vi "FestoCPX.Valve(2out2in).vi"(4 "Delay [ms] (0)":u32, 6 "Timeout [ms] (5000)":u32=5000, 8 "error in (no error)":errorcluster, 9 "Position":T3, 10 "Valve outputs":T1[](array[typedef]), 11 "Inputs":T2[](array[typedef])) -> (0 "error out":errorcluster, 2 "Aborted?":bool, 3 "Timeout?":bool)   [LabVIEW 2016]
uses:
  Station/Station.ValvePosition.ctl
  FestoCPX.DI.Signal.ctl
  FestoCPX.DO.Signal.ctl
  FestoCPX.DI.Data.State.Get.vi
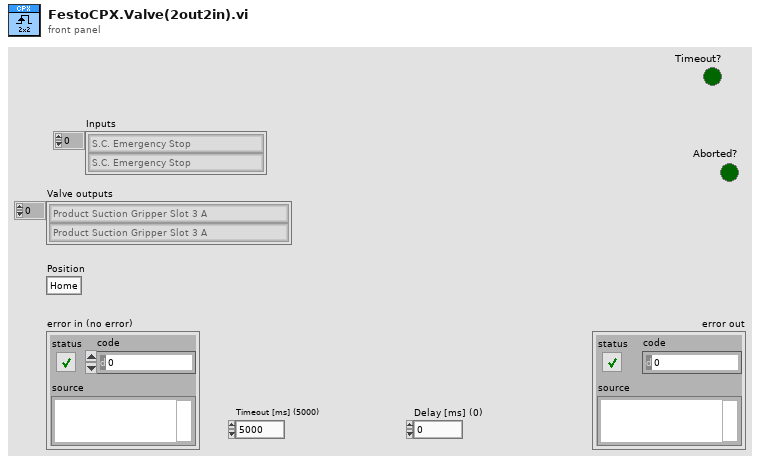
[diagram p1: front panel]
types:
  T1 = typedef "FestoCPX.DO.Signal.ctl" = enum16{"Safety Reset", "Air Main Valve", "Door Lock", "Button LED Start", "Button LED Stop", "Button LED Control", "Traffic LED Red", "Traffic LED Orange", "Traffic LED Green", "Horn", "Laser Interlock", "Laser Trigger", "Laser Fume Extractor", "Product Suction Gripper Slot 1 A", "Product Suction Gripper Slot 1 B", "Product Suction Gripper Slot 2 A", "Product Suction Gripper Slot 2 B", "Product Suction Gripper Slot 3 A", "Product Suction Gripper Slot 3 B", "Product Suction Gripper Slot 4 A", "Product Suction Gripper Slot 4 B", "Product Suction Gripper Final A", "Product Suction Gripper Final B", "Lamp", "Q1 Product Move Work", "Q1 Product Move Home", "Q2 Table Turn Work", "Q2 Table Turn Home", "Q3 Product Lift A", "Q3 Product Lift B", "Q4 Product Arm OK", "Q4 Product Arm NOK", "Q5 Product Arm Work", "Q6 Product BlowOut A", "Q6 Product BlowOut B"}
  T2 = typedef "FestoCPX.DI.Signal.ctl" = enum16{"S.C. Emergency Stop", "S.C. Side Door Close", "S.C. Front Door Close", "S.C. Front Door Secured", "Button Start", "Button Stop", "Button Control", "Product Move Home", "Product Move Work", "Table Position", "Table Lock", "Product Lift A Home", "Product Lift B Home", "Product Arm OK", "Product Arm NOK", "Product Arm Work", "Revolver ID 1", "Revolver ID 2", "Revolver ID 3", "Revolver ID 4", "Revolver ID 5", "Air Pressure Inside", "Air Pressure Inlet", "Product Slot 1 A Present", "Product Slot 1 B Present", "Product Slot 2 A Present", "Product Slot 2 B Present", "Product Slot 3 A Present", "Product Slot 3 B Present", "Product Slot 4 A Present", "Product Slot 4 B Present", "Product Final A Present", "Product Final B Present", "Product Output A Present", "Product Output B Present", "Product Container OK Present", "Product Container NOK Present", "Fork ID 1", "Fork ID 2"}
  T3 = typedef "Station.ValvePosition.ctl" = enum16{"Home", "Work"}
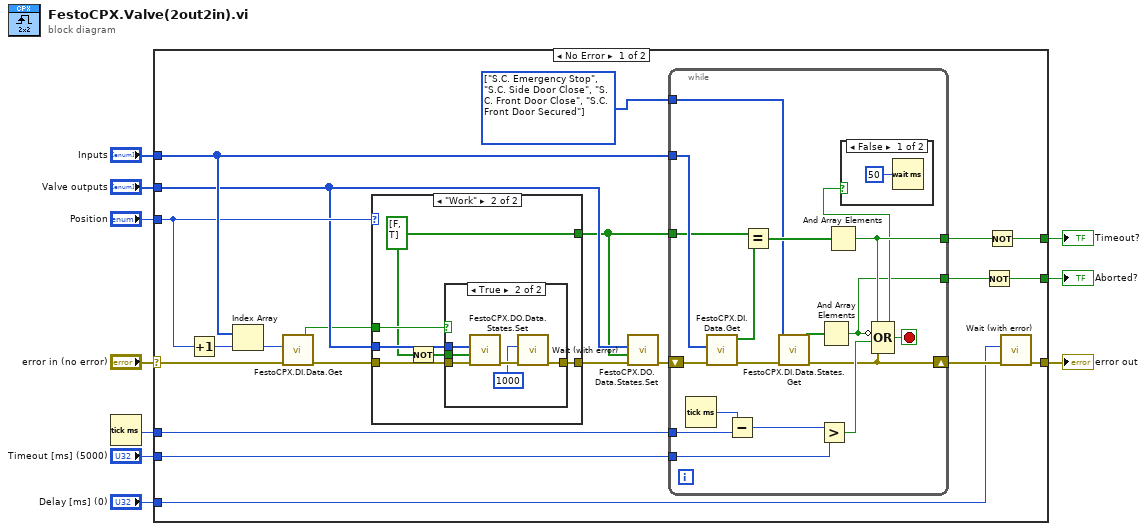
[diagram p0: block diagram]
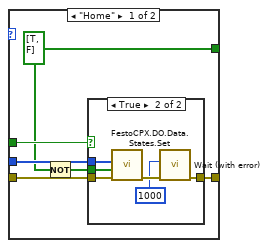
[diagram p3: hidden frame]
diagram:
  n1 = Tick Count (ms)() -> (millisecond timer value=w6:u32)
  n2 = case shown="No Error" "error in (no error)" {
    selector: "error in (no error)" -> [w23 w76]
    tunnel: "Position" -> [w20 _]
    tunnel: [w26 w76] -> w9
    tunnel: [w29 _] -> w8
    tunnel: w6 -> [w31 _]
    tunnel: "Timeout [ms] (5000)" -> [w30 _]
    tunnel: "Inputs" -> [w21 _]
    tunnel: "Valve outputs" -> [w18 _]
    tunnel: "Delay [ms] (0)" -> [w25 _]
    tunnel: [w12 _] -> w1
    frame No Error {
      w14 = T2[] [enum."S.C. Emergency Stop", enum."S.C. Side Door Close", enum."S.C. Front Door Close", enum."S.C. Front Door Secured"] items=["S.C. Emergency Stop", "S.C. Side Door Close", "S.C. Front Door Close", "S.C. Front Door Secured", "Button Start", "Button Stop", "Button Control", "Product Move Home", "Product Move Work", "Table Position", "Table Lock", "Product Lift A Home", "Product Lift B Home", "Product Arm OK", "Product Arm NOK", "Product Arm Work", "Revolver ID 1", "Revolver ID 2", "Revolver ID 3", "Revolver ID 4", "Revolver ID 5", "Air Pressure Inside", "Air Pressure Inlet", "Product Slot 1 A Present", "Product Slot 1 B Present", "Product Slot 2 A Present", "Product Slot 2 B Present", "Product Slot 3 A Present", "Product Slot 3 B Present", "Product Slot 4 A Present", "Product Slot 4 B Present", "Product Final A Present", "Product Final B Present", "Product Output A Present", "Product Output B Present", "Product Container OK Present", "Product Container NOK Present", "Fork ID 1", "Fork ID 2"] ("CPX.DI")
      n3 = Increment(x=w20) -> (x+1=w19:T3)
      n4 = Index Array(array=w21, index=w19) -> (element=w24:T2)
      n5 = call-poly "FestoCPX.DI.Data.Get.vi"("error in (no error)"=w23, "CPX.DI"=w24) -> ("error out"=w22:errorcluster, "State"=w11:bool)  [unwired: 5 in, 3 out]
      n6 = case shown="\"Work\"" w20 {
        tunnel: [w51 w64] -> w17
        tunnel: w22 -> [w55 w68]
        tunnel: w11 -> [w52 w65]
        tunnel: w18 -> [w53 w66]
        tunnel: [w54 w67] -> w16
        frame "Home" {
          w51 = bool[] [TRUE, FALSE]
          n7 = Not(x=w51) -> (.not. x?=w50:bool[])
          n8 = case shown="True" w52 {
            tunnel: w55 -> [w56 w62]
            tunnel: [w56 w57] -> w54
            tunnel: w50 -> [_ w61]
            tunnel: w53 -> [_ w60]
            frame False {
            }
            frame True {
              n9 = call "FestoCPX.DO.Data.States.Set.vi"("error in (no error)"=w62, "State"=w61, "CPX.DO"=w60) -> ("error out"=w59:errorcluster)  [unwired: 8 in]
              n10 = call "Wait (with error).vi"("error in (no error)"=w59, "milliseconds to wait"=u32 1000 ("Delay [ms] (0)")) -> ("error out"=w57:errorcluster)  [unwired: 8 in, 1 out]
            }
          }
        }
        frame "Work" {
          w64 = bool[] [FALSE, TRUE]
          n11 = Not(x=w64) -> (.not. x?=w63:bool[])
          n12 = case shown="True" w65 {
            tunnel: w68 -> [w69 w73]
            tunnel: [w69 w70] -> w67
            tunnel: w63 -> [_ w72]
            tunnel: w66 -> [_ w71]
            frame False {
            }
            frame True {
              n13 = call "FestoCPX.DO.Data.States.Set.vi"("error in (no error)"=w73, "State"=w72, "CPX.DO"=w71) -> ("error out"=w75:errorcluster)  [unwired: 8 in]
              n14 = call "Wait (with error).vi"("error in (no error)"=w75, "milliseconds to wait"=u32 1000 ("Delay [ms] (0)")) -> ("error out"=w70:errorcluster)  [unwired: 8 in, 1 out]
            }
          }
        }
      }
      n15 = call "FestoCPX.DO.Data.States.Set.vi"("error in (no error)"=w16, "State"=w17, "CPX.DO"=w18) -> ("error out"=w15:errorcluster)  [unwired: 8 in]
      n16 = while {
        shift-right: [w36] -> w27
        shift-left: w15 -> [w48]
        tunnel: w21 -> [w47]
        tunnel: [w39] -> w28
        tunnel: w31 -> [w45]
        tunnel: w30 -> [w43]
        tunnel: w17 -> [w42]
        tunnel: w14 -> [w35]
        tunnel: [w34] -> w13
        stop <- w38 stop-if-true
        n17 = Tick Count (ms)() -> (millisecond timer value=w46:u32)
        n18 = call-poly "FestoCPX.DI.Data.Get.vi"("error in (no error)"=w48, "CPX.DI"=w47) -> ("error out"=w37:errorcluster, "State"=w32:bool[])  [unwired: 5 in, 3 out]
        n19 = Subtract(x=w46, y=w45) -> (x-y=w44:u32)
        n20 = Equal?(x=w42, y=w32) -> (x = y?=w41:bool[])
        n21 = call "FestoCPX.DI.Data.States.Get.vi"("error in (no error)"=w37, "CPX.DI"=w35) -> ("error out"=w36:errorcluster, "State"=w33:bool[])  [unwired: 5 in, 3 out]
        n22 = Greater?(x=w44, y=w43) -> (0:w40:bool)
        n23 = And Array Elements(Boolean array=w33) -> (logical AND=w34:bool)
        n24 = And Array Elements(Boolean array=w41) -> (logical AND=w39:bool)
        n25 = Compound Arithmetic op=OR(w39, invert w34, w40, w36) -> (w38:bool)
        n26 = case shown="False" w38 {
          frame False {
            n27 = Wait (ms)(milliseconds to wait=u32 50) -> ()  [unwired: 1 out]
          }
          frame True {
          }
        }
      }
      n28 = Not(x=w13) -> (.not. x?=w12:bool)
      n29 = Not(x=w28) -> (.not. x?=w29:bool)
      n30 = call "Wait (with error).vi"("error in (no error)"=w27, "milliseconds to wait"=w25) -> ("error out"=w26:errorcluster)  [unwired: 8 in, 1 out]
    }
    frame Error {
    }
  }
  "error out" <- w9
  "Timeout?" <- w8
  "Aborted?" <- w1
